vi "niDTS BT Rx Test UTIL BT TX Parameters to LE Parameters.vi"(7 "BT Tx Parameters":T6={"Channel"=1, "Dut Tx Power"=0.0, "External Attenuation (dB)"=[0.0], "Data Rate"=enum."3", "Packet type"=enum."DH1", "Payload Data"=enum."PN9", "Carrier Mode"=enum."Burst", "Number of Packets"=2, "Report Period (ms)"=0.0, "BD ADDRESS"=12329017, "Dirty Tx"=FALSE, "Corrupt Alternate CRC"=FALSE, "Packet Header"={"LT Address"=0, "Flow"=3, "ARQN"=enum."NAK", "Sequence Bit"=0}, "Payload Header"={"LCh"=0, "HeaderFlowControlBit"=FALSE, "Length (-1 AutoSet Max)"=0}, "Trigger"={"TriggerEdge"=enum."RISing", "TriggerSource"=enum."RTSI 0", "TriggerDelay (sec)"=0.0, "TriggerTimeout (sec)"=0.00015}} {"BD ADDRESS" max=16777215 format="%.0x"}) -> (8 "BT BDR Parameters":T1={"Channel"=0, "Tx Power (dBm)"=0.0, "External Attenuation (dB)"=0.0, "Payload Data"=enum."00001111", "Carrier Mode"=enum."Burst", "Number of Packets"=4, "Corrupt Alternate CRC"=FALSE, "Dirty Tx"=FALSE, "Payload Header"={"Length (-1 AutoSet Max)"=0}, "Trigger"={"TriggerEdge"=enum."RISing", "TriggerSource"=enum."IMMediate", "TriggerDelay (sec)"=0.0, "TriggerTimeout (sec)"=0.0}})   [LabVIEW 2014, in "niDTS BT.lvlib"]
uses:
  niDTS BT.lvlib
  Rx Test/Includes/niDTS BT Rx Test INC Parameters.ctl
  Includes/niDTS BT INC Packet Type.ctl
  Tx Test/Includes/niDTS BT Tx Test INC BD Payload Data.ctl
  Rx Test/Includes/niDTS BT Rx Test INC Carrier Mode.ctl
  Rx Test/Includes/niDTS BT Rx Test INC Packet Header.ctl
  Rx Test/Includes/niDTS BT Rx Test INC Payload Header.ctl
  Includes/niDTS BT DUT INC SG Trigger.ctl
  Includes/niDTS BT LE Rx Test INC Parameters.ctl
  Rx Test/Includes/niDTS BT Rx Test INC LE Payload Length.ctl
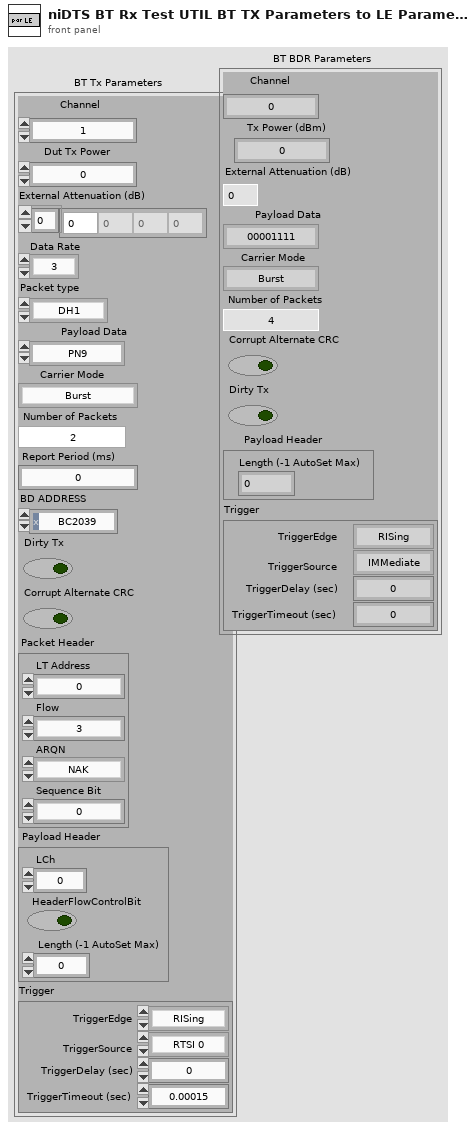
[diagram p1: front panel]
types:
  T1 = typedef "niDTS BT.lvlib/niDTS BT LE Rx Test INC Parameters.ctl" = cluster{"Channel":i32, "Tx Power (dBm)":dbl, "External Attenuation (dB)":dbl, "Payload Data":T2, "Carrier Mode":T3, "Number of Packets":i32, "Corrupt Alternate CRC":bool, "Dirty Tx":bool, "Payload Header":T4, "Trigger":T5}
  T2 = typedef "niDTS BT.lvlib/niDTS BT Tx Test INC BD Payload Data.ctl" = enum16{"0", "1", "01", "00001111", "PN9", "AUTO"}
  T3 = typedef "niDTS BT.lvlib/niDTS BT Rx Test INC Carrier Mode.ctl" = enum16{"Burst", "Continuous"}
  T4 = typedef "niDTS BT.lvlib/niDTS BT Rx Test INC LE Payload Length.ctl" = cluster{"Length (-1 AutoSet Max)":i32}
  T5 = typedef "niDTS BT.lvlib/niDTS BT DUT INC SG Trigger.ctl" = cluster{"TriggerEdge":enum16{"RISing", "FALLing"}, "TriggerSource":enum16{"IMMediate", "PFI 0", "PFI 1", "RTSI 0", "RTSI 1", "RTSI 2", "RTSI 3", "RTSI 4", "RTSI 5", "RTSI 6", "RTSI 7", "PXI STAR", "Software"}, "TriggerDelay (sec)":dbl, "TriggerTimeout (sec)":dbl}
  T6 = typedef "niDTS BT.lvlib/niDTS BT Rx Test INC Parameters.ctl" = cluster{"Channel":i32, "Dut Tx Power":dbl, "External Attenuation (dB)":dbl[], "Data Rate":enum16{"1", "2", "3"}, "Packet type":T7, "Payload Data":T2, "Carrier Mode":T3, "Number of Packets":i32, "Report Period (ms)":dbl, "BD ADDRESS":i64, "Dirty Tx":bool, "Corrupt Alternate CRC":bool, "Packet Header":T8, "Payload Header":T9, "Trigger":T5}
  T7 = typedef "niDTS BT.lvlib/niDTS BT INC Packet Type.ctl" = enum16{"NULL", "POLL", "FHS", "DM1", "DH1", "HV1", "HV2", "HV3", "EV3", "DV", "AUX1", "DM3", "DH3", "EV4", "EV5", "DM5", "DH5", "LE-TP"}
  T8 = typedef "niDTS BT.lvlib/niDTS BT Rx Test INC Packet Header.ctl" = cluster{"LT Address":i8, "Flow":i8, "ARQN":enum16{"NAK", "ACK"}, "Sequence Bit":i8}
  T9 = typedef "niDTS BT.lvlib/niDTS BT Rx Test INC Payload Header.ctl" = cluster{"LCh":i32, "HeaderFlowControlBit":bool, "Length (-1 AutoSet Max)":i32}
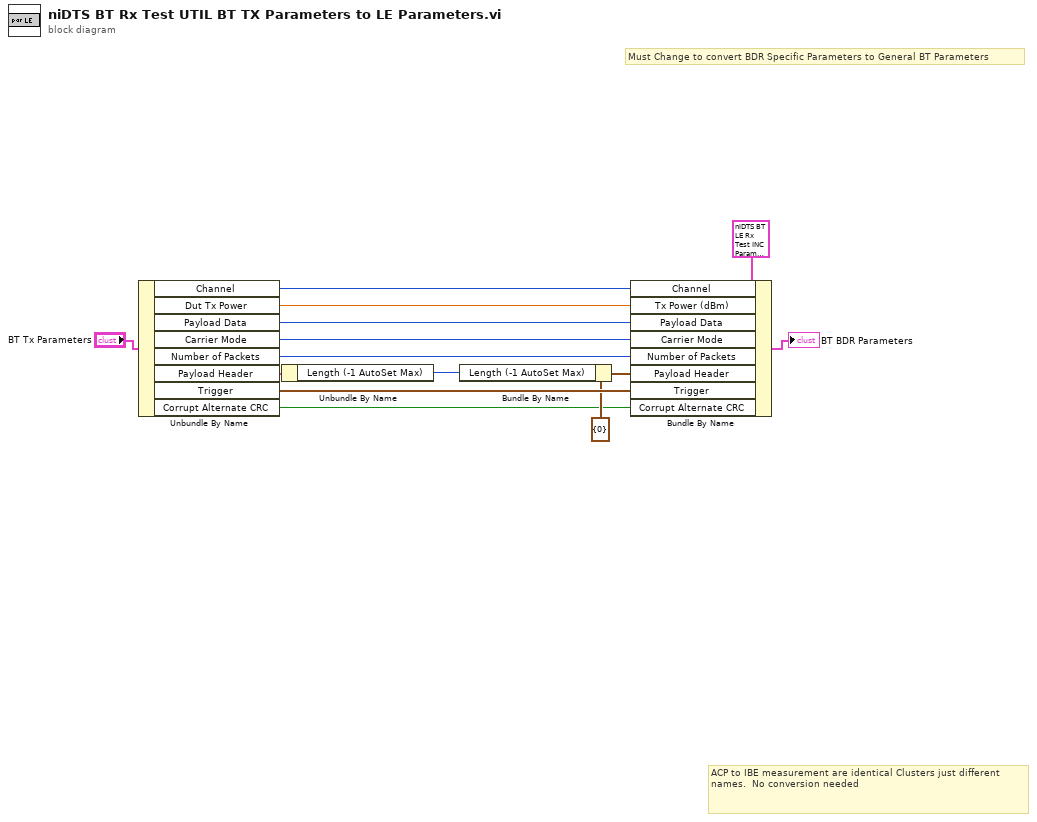
[diagram p0: block diagram]
diagram:
  # "ACP to IBE measurement are identical Clusters just different names.  No conversion needed"
  # "Must Change to convert BDR Specific Parameters to General BT Parameters"
  n1 = Unbundle By Name("BT Tx Parameters") -> ("Channel"=w13:i32, "Dut Tx Power"=w2:dbl, "Payload Data"=w12:T2, "Carrier Mode"=w11:T3, "Number of Packets"=w10:i32, "Payload Header"=w8:T9, "Trigger"=w9:T5, "Corrupt Alternate CRC"=w1:bool)
  n2 = Unbundle By Name(w8) -> ("Length (-1 AutoSet Max)"=w6:i32)
  n3 = Bundle By Name(cluster=T4 {"Length (-1 AutoSet Max)"=0} ("Payload Header"), "Length (-1 AutoSet Max)"=w6) -> (w5:T4)
  n4 = Bundle By Name(cluster=T1 {"Channel"=0, "Tx Power (dBm)"=0.0, "External Attenuation (dB)"=0.0, "Payload Data"=enum."00001111", "Carrier Mode"=enum."Burst", "Number of Packets"=4, "Corrupt Alternate CRC"=FALSE, "Dirty Tx"=FALSE, "Payload Header"={"Length (-1 AutoSet Max)"=0}, "Trigger"={"TriggerEdge"=enum."RISing", "TriggerSource"=enum."IMMediate", "TriggerDelay (sec)"=0.0, "TriggerTimeout (sec)"=0.0}} ("BT BDR Parameters"), "Channel"=w13, "Tx Power (dBm)"=w2, "Payload Data"=w12, "Carrier Mode"=w11, "Number of Packets"=w10, "Payload Header"=w5, "Trigger"=w9, "Corrupt Alternate CRC"=w1) -> (→"BT BDR Parameters":T1)
